vi "Initialize.vi"(8 "error in":errorcluster, 11 "Plugin in":refnum<class "StreamReader.lvclass">) -> (0 "error out":errorcluster, 3 "Plugin out":refnum<class "StreamReader.lvclass">)   [LabVIEW 2024, in "StreamReader.lvlib" / "StreamReader.lvclass"]
uses:
  StreamReader.lvclass
  StreamReader Parameters.ctl
  <vilib>/FlexLogger/SDK/PluginSDK.lvlibp/PEFClasses/SDK/Processing Element/Timing Parameters.ctl
  <vilib>/FlexLogger/SDK/PluginSDK.lvlibp/PEFClasses/SDK/Processing Element/Timing Method.ctl
  StreamReader.lvclass/StreamReader.ctl
  StreamReader Strings.vi
  <vilib>/FlexLogger/SDK/PluginSDK.lvlibp/PEFClasses/SDK/Plugin/ParameterAccess/Write String.vi
  <vilib>/FlexLogger/SDK/PluginSDK.lvlibp/PEFClasses/SDK/Plugin/ParameterAccess/Write I32.vi
  <vilib>/FlexLogger/SDK/PluginSDK.lvlibp/PEFClasses/SDK/Plugin/Plugin.lvclass
  <vilib>/FlexLogger/SDK/PluginSDK.lvlibp/PEFClasses/SDK/Processing Element/Processing Element.lvclass
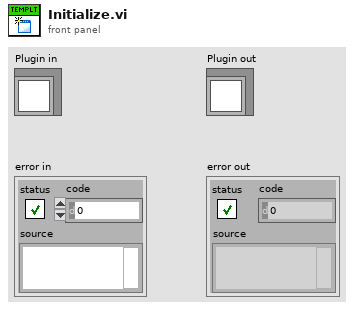
[diagram p1: front panel]
types:
  T1 = typedef "PluginSDK.lvlibp/Processing Element.lvclass/Timing Parameters.ctl" = cluster{"Timing Method":T2, "Timing Period (ms)":i32}
  T2 = typedef "PluginSDK.lvlibp/Processing Element.lvclass/Timing Method.ctl" = enum16{"Periodic", "Immediate", "On Data Ready", "Triggered"}
  T3 = typedef "StreamReader.lvlib/StreamReader.lvclass/StreamReader Parameters.ctl" = cluster{"Reader URL":string, "Writer URL":string, "Timeout":i32, "Buffer Size":i32, "Reader endpoint":refnum<k21>, "Channel Names":string[]}
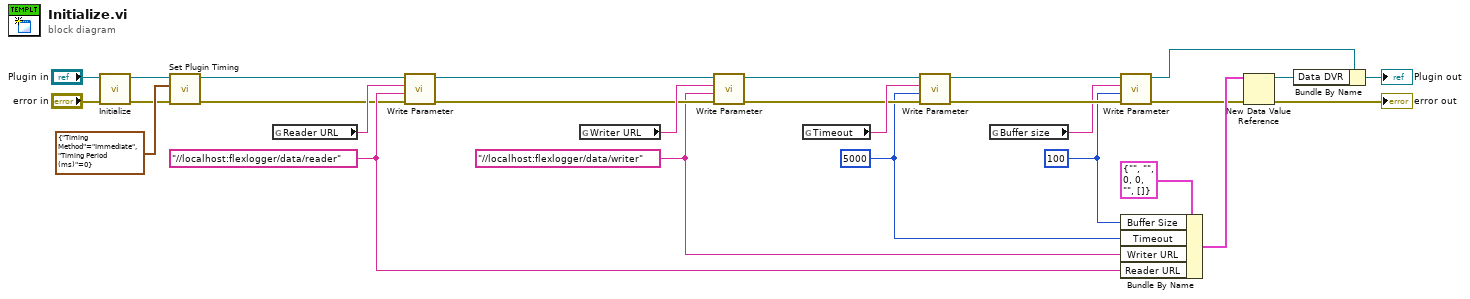
[diagram p0: block diagram]
diagram:
  w11 = "//localhost:flexlogger/data/reader" ("Value")
  w9 = 5000 ("Value")
  w8 = 100 ("Value")
  w10 = "//localhost:flexlogger/data/writer" ("Value")
  n1 = call-parent "Initialize.vi"("error in (no error)"="error in", "Plugin in"="Plugin in") -> ("error out"=w2:errorcluster, "Plugin out"=w4:refnum<class "StreamReader.lvclass">)  [unwired: 8 in]
  n2 = call <vilib>:"Set Plugin Timing.vi"("error in (no error)"=w2, "Timing Parameters"=T1 {"Timing Method"=enum."Immediate", "Timing Period (ms)"=0}, "Plugin in"=w4) -> ("error out"=w1:errorcluster, "Plugin out"=w3:refnum<class "StreamReader.lvclass">)  [unwired: 7 in]
  n3 = global read "StreamReader Strings.vi" "Reader URL"() -> (w21:string)
  n4 = call-poly <vilib>:"Write Parameter.vi"("error in (no error)"=w1, "Value"=w11, "Name"=w21, "Plugin in"=w3) -> ("error out"=w19:errorcluster, "Plugin out"=w20:refnum<class "StreamReader.lvclass">)  [unwired: 6 in]
  n5 = global read "StreamReader Strings.vi" "Writer URL"() -> (w24:string)
  n6 = call-poly <vilib>:"Write Parameter.vi"("error in (no error)"=w19, "Value"=w10, "Name"=w24, "Plugin in"=w20) -> ("error out"=w17:errorcluster, "Plugin out"=w18:refnum<class "StreamReader.lvclass">)  [unwired: 6 in]
  n7 = global read "StreamReader Strings.vi" "Timeout"() -> (w22:string)
  n8 = call-poly <vilib>:"Write Parameter.vi"("error in (no error)"=w17, "Value"=w9, "Name"=w22, "Plugin in"=w18) -> ("error out"=w25:errorcluster, "Plugin out"=w26:refnum<class "StreamReader.lvclass">)  [unwired: 6 in]
  n9 = global read "StreamReader Strings.vi" "Buffer size"() -> (w23:string)
  n10 = call-poly <vilib>:"Write Parameter.vi"("error in (no error)"=w25, "Value"=w8, "Name"=w23, "Plugin in"=w26) -> ("error out"=w7:errorcluster, "Plugin out"=w15:refnum<class "StreamReader.lvclass">)  [unwired: 6 in]
  n11 = Bundle By Name(cluster=T3 {"Reader URL"="", "Writer URL"="", "Timeout"=0, "Buffer Size"=0, "Reader endpoint"="", "Channel Names"=[]} ("StreamReader Parameters"), "Buffer Size"=w8, "Timeout"=w9, "Writer URL"=w10, "Reader URL"=w11) -> (w12:T3)
  n12 = New Data Value Reference(data value=w12, error in=w7) -> (data value reference=w16:refnum<data-value>, error out=→"error out":errorcluster)
  n13 = Bundle By Name(cluster=w15, "Data DVR"=w16) -> (→"Plugin out":refnum<class "StreamReader.lvclass">)
